vi "Temperature Reading with add shifter.vi"() -> ()   [LabVIEW 2020]
panel:
  out "Index MIN":dbl
  out "Index MAX":dbl
  out "Temp MIN":dbl
  out "Temp MAX":dbl
  out "WARNING":bool
  in  "stop":bool
  out "Waveform Chart":T1(graph)
  in  "LOW Limit":dbl
  in  "HIGH Limit":dbl
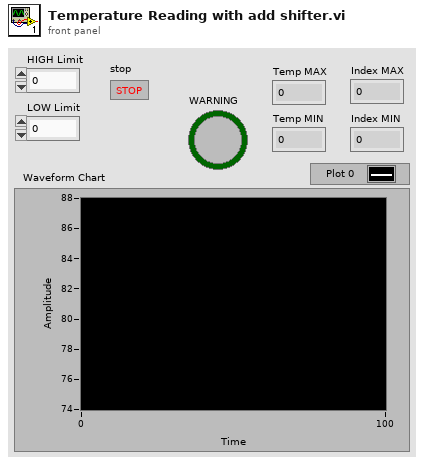
[diagram p1: front panel]
types:
  T1 = cluster{"HIGH Limit":dbl, "Temperature (deg F)":dbl, "LOW Limit":dbl}
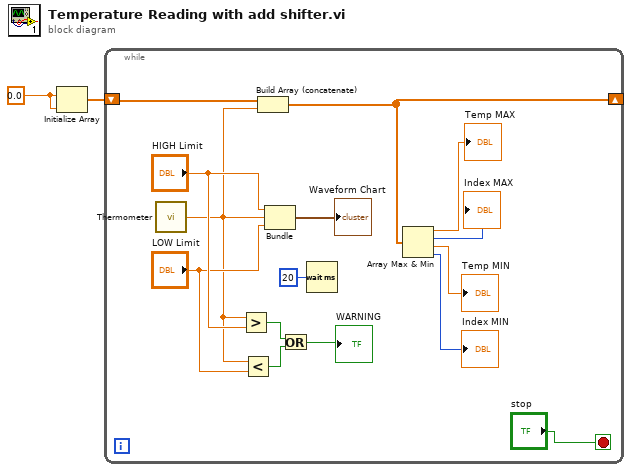
[diagram p0: block diagram]
diagram:
  w2 = 0.0 ("element")
  n1 = Initialize Array "Initialize Array"(w2, w2) -> (w1:dbl[])
  n2 = while {
    shift-right: [w3] -> _
    shift-left: w1 -> [w9]
    stop <- "stop" stop-if-true
    n3 = call "Thermometer.vi"() -> ("Temperature (deg F)"=w8:dbl)  [unwired: 1 in]
    n4 = Greater?(x=w8, y="HIGH Limit") -> (0:w14:bool)
    n5 = Less?(x=w8, y="LOW Limit") -> (x < y?=w13:bool)
    n6 = Build Array (concatenate) "Build Array"(w9, w8) -> (w3:dbl[])
    n7 = Bundle("HIGH Limit"="HIGH Limit", "Temperature (deg F)"=w8, "LOW Limit"="LOW Limit") -> (→"Waveform Chart":T1)  [unwired: 1 in]
    n8 = Or(x=w14, y=w13) -> (x .or. y?=→"WARNING":bool)
    n9 = Wait (ms)(milliseconds to wait=u32 20) -> ()  [unwired: 1 out]
    n10 = Array Max & Min(array=w3) -> (max value=→"Temp MAX":dbl, max index (indices)=→"Index MAX":i32, min value=→"Temp MIN":dbl, min index (indices)=→"Index MIN":i32)
  }
